vi "BitAtPosition.vi"(8 "Error In":errorcluster, 10 "p":i32, 11 "n":i32) -> (0 "Error Out":errorcluster, 3 "Value":i16)   [LabVIEW 2020, in "LiFingerprint.lvclass"]
uses:
  LiFingerprint.lvclass
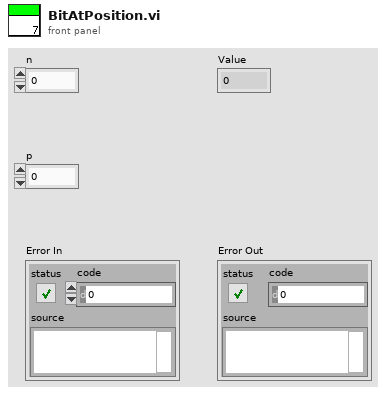
[diagram p1: front panel]
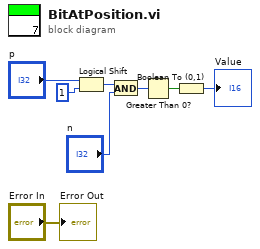
[diagram p0: block diagram]
diagram:
  n1 = Logical Shift(y="p", x=u32 1) -> (x << y=w6:u32)
  n2 = And(x=w6, y="n") -> (x .and. y?=w4:u32)
  n3 = Greater Than 0?(x=w4) -> (x > 0?=w3:bool)
  n4 = Boolean To (0,1)(Boolean=w3) -> (0, 1=→"Value":i16)
  "Error Out" <- "Error In"
